vi "Do.vi"(8 "error in (no error)":errorcluster, 10 "Rival":refnum<class "Peasant.lvclass">, 11 "Accessory in":refnum<class "Accessory.lvclass">) -> (0 "error out":errorcluster, 2 "Rival":refnum<class "Peasant.lvclass">, 3 "Accessory out":refnum<class "Accessory.lvclass">)   [LabVIEW 2021, in "Accessory.lvclass"]
uses:
  Accessory.lvclass
  Peasant/Peasant.lvclass
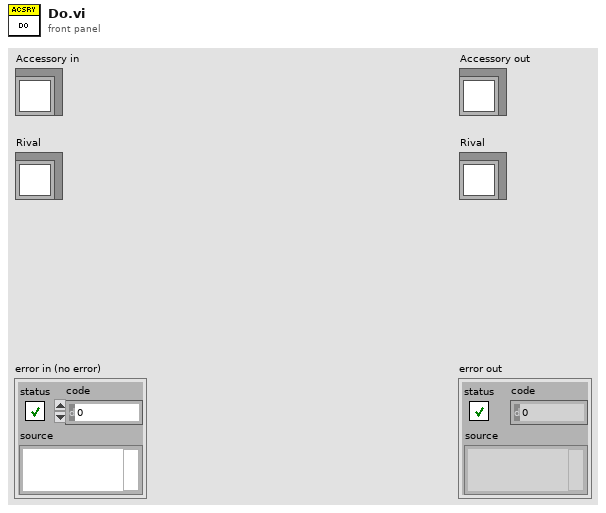
[diagram p1: front panel]
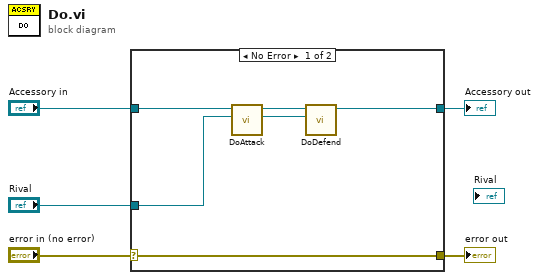
[diagram p0: block diagram]
diagram:
  n1 = case shown="No Error" "error in (no error)" {
    selector: "error in (no error)" -> [w11 w13]
    tunnel: [w11 w13] -> w4
    tunnel: [w8 w12] -> w2
    tunnel: "Accessory in" -> [w9 w12]
    tunnel: "Rival" -> [w7 _]
    frame No Error {
      n2 = call-dynamic "DoAttack.vi"("Rival"=w7, "Accessory in"=w9) -> ("Rival"=w6:refnum<class "Peasant.lvclass">, "Accessory out"=w10:refnum<class "Accessory.lvclass">)  [unwired: 7 in, 1 out]
      n3 = call-dynamic "DoDefend.vi"("Rival"=w6, "Accessory in"=w10) -> ("Accessory out"=w8:refnum<class "Accessory.lvclass">)  [unwired: 7 in, 2 out]
    }
    frame Error {
    }
  }
  "error out" <- w4
  "Accessory out" <- w2
